vi "Defect detection after UV.vi"(8 "error in (no error)":errorcluster, 10 "Fiber Auto Collimation state data in":refnum<class "Fiber Auto Collimation state data.lvclass">, 11 "Station config in":refnum<class "Station config.lvclass">) -> (0 "error out":errorcluster, 2 "Fiber Auto Collimation state data out":refnum<class "Fiber Auto Collimation state data.lvclass">, 3 "Station config out":refnum<class "Station config.lvclass">)   [LabVIEW 2018]
uses:
  State data/Fiber Auto Collimation state data.lvclass
  <userlib>/Recipe/Station Config/Station config.lvclass
  <userlib>/nLight Tidbits/Logging/Controls/Logging type choice.ctl
  State data/Fiber Auto Collimation state data.lvclass/Fiber Auto Collimation state data.ctl
  <instrlib>/nLight Instruments/Motion Controller/Axis index.ctl
  State data/Add Changed data.vi
  <instrlib>/nLight Instruments/Beam Profiler/Beam Profiler.lvclass
  <instrlib>/nLight Instruments/Motion Controller/Motion Controller.lvclass
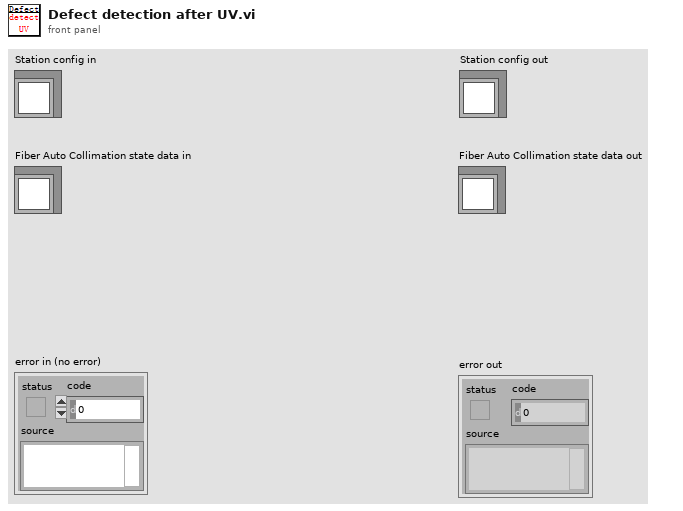
[diagram p1: front panel]
types:
  T1 = typedef "Logging type choice.ctl" = enum16{"No log type selected", "Testing start/stop", "Test progress", "Station startup/shutdown", "Station config change", "Recipe load/change", "Inventory transaction", "Instrument", "Debug"}
  T2 = typedef "Test Parameters.ctl" = cluster{"Start position":dbl, "Peak Resp_min":dbl, "Circularity_min":dbl, "Beam Size Target":dbl, "Beam Size Percentage ":dbl, "Collimation Steps Data Path":string, "Collimation Data Path":string, "Defect detection Image Path":string, "Save Collimation Steps Data Enable":bool, "Defect detection Enable":bool, "Stop position":dbl}
  T3 = typedef "Fiber Auto Collimation state data.lvclass/BV Data.ctl" = cluster{"Centroid X[um]":sgl, "Centroid Y[um]":sgl, "PeakResp.[%]":dbl, "Knife Edge X[mm]":sgl, "Knife Edge Y[mm]":sgl, "Circularity":sgl, "Collimation Result":bool}
  T4 = typedef "IMAQ Image.ctl" = refnum<image>
  T5 = typedef "VBAIInterface.ctl" = refnum<k21>
  T6 = typedef "Motion Controller.lvclass/Axis index.ctl" = i32
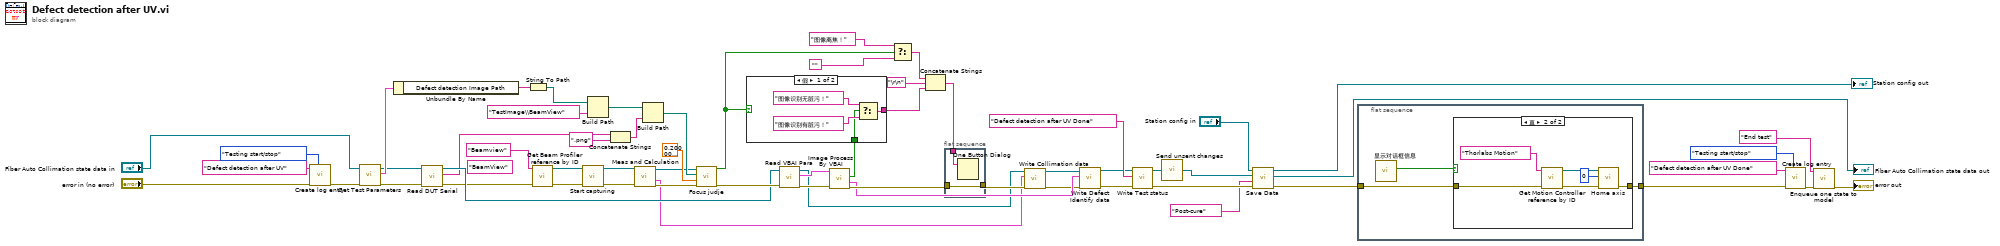
[diagram p0: block diagram]
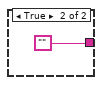
[diagram p2: hidden frame]
diagram:
  (unwired) "BeamView"
  n1 = call <userlib>:"Create log entry.vi"("Logging type choice"=Logging_type_choice."Testing start/stop", "error in (no error)"="error in (no error)", "Brief log entry"="Defect detection after UV") -> ("error out"=w37:errorcluster)  [unwired: 8 in]
  n2 = call "Get Test Parameters.vi"("error in (no error)"=w37, "Fiber Auto Collimation state data in"="Fiber Auto Collimation state data in") -> ("error out"=w59:errorcluster, "TestParameters"=w61:T2, "Fiber Auto Collimation state data out"=w60:refnum<class "Fiber Auto Collimation state data.lvclass">)  [unwired: 7 in]
  n3 = Unbundle By Name(w61) -> ("Defect detection Image Path"=w50:string)
  n4 = call "Read DUT Serial.vi"("error in (no error)"=w59, "Fiber Auto Collimation state data in"=w60) -> ("error out"=w18:errorcluster, "DUT Serial"=w51:string, "Fiber Auto Collimation state data out"=w52:refnum<class "Fiber Auto Collimation state data.lvclass">)  [unwired: 7 in]
  n5 = String To Path(string=w50) -> (path=w57:path)
  n6 = call <instrlib>:"Get Beam Profiler reference by ID.vi"("error in (no error)"=w18, "Identifier"="Beamview") -> ("error out"=w22:errorcluster, "Beam Profiler out"=w21:refnum<class "Beam Profiler.lvclass">)  [unwired: 8 in]
  n7 = call-dynamic "Start capturing.vi"("error in (no error)"=w22, "Beam Profiler in"=w21) -> ("error out"=w15:errorcluster, "Beam Profiler out"=w16:refnum<class "Beam Profiler.lvclass">)  [unwired: 8 in]
  n8 = Build Path(base path=w57, name or relative path="TestImage\\BeamView") -> (appended path=w54:path)
  n9 = Concatenate Strings(w51, ".png" ("string")) -> (w55:string)
  n10 = call "Meas and Calculation.vi"("error in (no error)"=w15, "Beam Profiler in"=w16) -> ("error out"=w14:errorcluster, "BV Data"=w8:T3, "Beam Profiler out"=w13:refnum<class "Beam Profiler.lvclass">)  [unwired: 6 in, 1 out]
  n11 = Build Path(base path=w54, name or relative path=w55) -> (appended path=w19:path)
  n12 = call "Focus judje.vi"("error in"=w14, "Standard Variation Limit"=sgl 0.2, "File Path"=w19, "Beam Profiler in"=w13) -> ("error out"=w53:errorcluster, "离焦？"=w23:bool)  [unwired: 5 in, 1 out]
  n13 = call "Read VBAI Para.vi"("error in (no error)"=w53, "Fiber Auto Collimation state data in"=w52) -> ("error out"=w27:errorcluster, "VBAI"=w26:cluster{"New Image":T4, "VBAI Session Out":T5}, "Fiber Auto Collimation state data out"=w10:refnum<class "Fiber Auto Collimation state data.lvclass">)  [unwired: 7 in]
  n14 = call "Image Process By VBAI.vi"("error in"=w27, "VBAI"=w26) -> ("error out"=w28:errorcluster, "Defect identify data"=w25:cluster{"Image":T4, "Measure Report":string}, "Result"=w24:bool)  [unwired: 4 in, 3 out]
  n15 = case shown="假" w23 {
    tunnel: [w63 ""] -> w41
    tunnel: w24 -> [w62 _]
    frame False {
      n16 = Select(t="图像识别无脏污！", s=w62, f="图像识别有脏污！") -> (s? t:f=w63:string)
    }
    frame True {
    }
  }
  n17 = Select(t="图像离焦！", s=w23, f="") -> (s? t:f=w43:string)
  n18 = Concatenate Strings(w43, "\r\n", w41) -> (w45:string)
  n19 = flat-sequence {
    tunnel: w28 -> [w68]
    tunnel: [w68] -> w11
    tunnel: w45 -> [w67]
    frame #0 {
      n20 = One Button Dialog(message=w67) -> ()  [unwired: 1 in, 1 out]
    }
  }
  n21 = call "Write Collimation data.vi"("error in (no error)"=w11, "BV Data"=w8, "Fiber Auto Collimation state data in"=w10) -> ("error out"=w12:errorcluster, "Fiber Auto Collimation state data out"=w9:refnum<class "Fiber Auto Collimation state data.lvclass">)  [unwired: 7 in]
  n22 = call "Write Defect Identify data.vi"("error in (no error)"=w12, "Defect Identify data"=w25, "Fiber Auto Collimation state data in"=w9) -> ("error out"=w47:errorcluster, "Fiber Auto Collimation state data out"=w46:refnum<class "Fiber Auto Collimation state data.lvclass">)  [unwired: 7 in]
  n23 = call "Write Test status.vi"("error in (no error)"=w47, "Test status"="Defect detection after UV Done", "Fiber Auto Collimation state data in"=w46) -> ("error out"=w7:errorcluster, "Fiber Auto Collimation state data out"=w49:refnum<class "Fiber Auto Collimation state data.lvclass">)  [unwired: 7 in]
  n24 = call "Send unsent changes.vi"("Fiber Auto Collimation state data in"=w49) -> ("Fiber Auto Collimation state data out"=w5:refnum<class "Fiber Auto Collimation state data.lvclass">)  [unwired: 1 in]
  n25 = call "Save Data.vi"("error in (no error)"=w7, "Process Sub Step"="Post-cure", "Fiber Auto Collimation state data in"=w5, "Station config in"="Station config in") -> ("error out"=w6:errorcluster, "Fiber Auto Collimation state data out"=→"Fiber Auto Collimation state data out":refnum<class "Fiber Auto Collimation state data.lvclass">, "Station config out"=→"Station config out":refnum<class "Station config.lvclass">)  [unwired: 5 in]
  n26 = flat-sequence {
    tunnel: w6 -> [w71]
    tunnel: [w70] -> w29
    frame #0 {
      n27 = call "显示对话框信息"() -> ("确定"=w69:bool)  [unwired: 10 in, 1 out]
      n28 = case shown="真" w69 {
        tunnel: w71 -> [w72 w75]
        tunnel: [w72 w77] -> w70
        frame False {
        }
        frame True {
          n29 = call <instrlib>:"Get Motion Controller reference by ID.vi"("error in (no error)"=w75, "Identifier"="Thorlabs Motion") -> ("error out"=w74:errorcluster, "Motion Controller out"=w73:refnum<class "Motion Controller.lvclass">)  [unwired: 8 in]
          n30 = call-dynamic "Home axis.vi"("error in (no error)"=w74, "Axis index"=T6 0, "Motion Controller in"=w73) -> ("error out"=w77:errorcluster)  [unwired: 7 in, 1 out]
        }
      }
    }
  }
  n31 = call <userlib>:"Create log entry.vi"("Logging type choice"=Logging_type_choice."Testing start/stop", "error in (no error)"=w29, "Brief log entry"="Defect detection after UV Done") -> ("error out"=w32:errorcluster)  [unwired: 8 in]
  n32 = call "Enqueue one state to model.vi"("error in (no error)"=w32, "Enqueued state"="End test") -> ("error out"=→"error out":errorcluster)  [unwired: 9 in]
